vi "Query Over Temperature Protection Status.vi"(8 "error in (no error)":errorcluster, 11 "VISA resource name":refnum<visa-resource-name>) -> (0 "error out":errorcluster, 2 "Over Temperature?":bool, 3 "VISA resource name out":refnum<visa-resource-name>)   [LabVIEW 2010, in "Agilent U2722.lvlib"]
doc: "Returns the status of over voltage temperature protection."
uses:
  Agilent U2722.lvlib
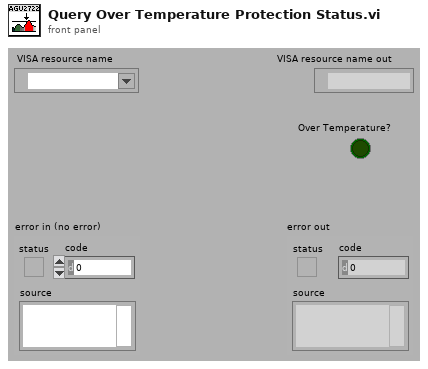
[diagram p1: front panel]
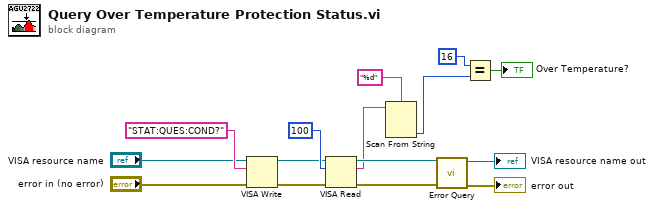
[diagram p0: block diagram]
diagram:
  n1 = VISA Write(VISA resource name="VISA resource name", write buffer="STAT:QUES:COND?", error in (no error)="error in (no error)") -> (VISA resource name out=w12:refnum<visa-resource-name>, error out=w11:errorcluster)  [unwired: 1 out]
  n2 = VISA Read(VISA resource name=w12, byte count=u32 100, error in (no error)=w11) -> (VISA resource name out=w8:refnum<visa-resource-name>, read buffer=w5:string, error out=w7:errorcluster)  [unwired: 1 out]
  n3 = Scan From String(format string="%d", input string=w5) -> (output 1=w3:i32)  [unwired: 3 in, 3 out]
  n4 = call "Error Query.vi"("error in (no error)"=w7, "VISA resource name"=w8) -> ("error out"=→"error out":errorcluster, "VISA resource name out"=→"VISA resource name out":refnum<visa-resource-name>)  [unwired: 6 in, 2 out]
  n5 = Equal?(x=16, y=w3) -> (x = y?=→"Over Temperature?":bool)
